vi "Configure Data Marker.vi"(8 "error in (no error)":errorcluster {"code" format="%.0x"}, 9 "DataMarker (Ss List Sequencer Setup Trigger Data Marker Marker1)":i32(ring) items=["Ss List Sequencer Setup Trigger Data Marker Marker1", "Ss List Sequencer Setup Trigger Data Marker Marker2", "Ss List Sequencer Setup Trigger Data Marker Marker3", "Ss List Sequencer Setup Trigger Data Marker Marker4"], 11 "instrument handle":refnum<k15>) -> (0 "error out":errorcluster {"code" format="%.0x"}, 3 "instrument handle out":refnum<k15>)   [LabVIEW 2009, in "Keysight XSAn.lvlib"]
doc: "Configure the output trigger maker routing to Marker for DataMarker in the whole source sequence.\n\nSupported Models: M8920A, M9420A, M9421A."
uses:
  <instrlib>/Keysight XSAn/Keysight XSAn.lvlib
  AgXSAn.dll
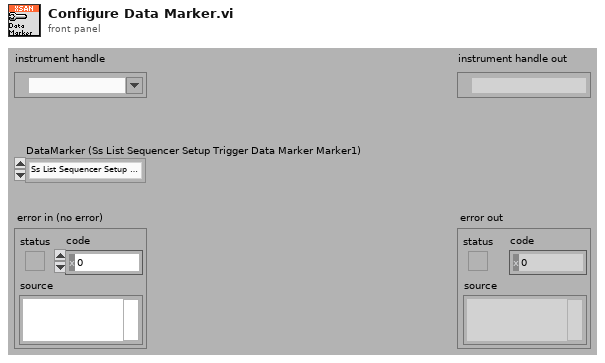
[diagram p1: front panel]
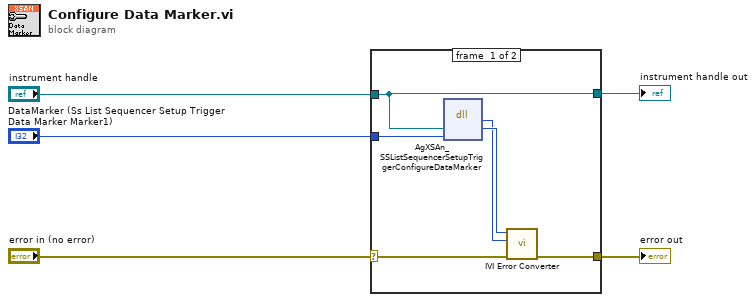
[diagram p0: block diagram]
diagram:
  n1 = case shown="No Error" "error in (no error)" {
    selector: "error in (no error)" -> [w9 w13]
    tunnel: [w8 w13] -> w5
    tunnel: "instrument handle" -> [w6 w12]
    tunnel: "DataMarker (Ss List Sequencer Setup Trigger Data Marker Marker1)" -> [w7 _]
    tunnel: [w6 w12] -> w1
    frame #0 {
      n2 = dll-call lib="AgXSAn**.dll" fn="AgXSAn_SSListSequencerSetupTriggerConfigureDataMarker"("Vi"=w6, "DataMarker"=w7) -> (w10:i32, "Vi"=w11:u32)  [unwired: 4 in, 2 out]
      n3 = call <instrlib>:"IVI Error Converter.vi"("error in (no error)"=w9, "IVI error code (0)"=w10, "instrument handle"=w11) -> ("error out"=w8:errorcluster)  [unwired: 7 in, 1 out]
    }
    frame #1 {
    }
  }
  "error out" <- w5
  "instrument handle out" <- w1
